vi "After Hook.vi"(8 "Error In":errorcluster, 11 "Hook VI In":path=path "") -> (0 "Error Out":errorcluster, 3 "Hook VI Out":path)   [LabVIEW 2018, in "Tests.lvlib" / "Toolkit.lvlib" / "Integration.lvlib"]
uses:
  Integration.lvlib
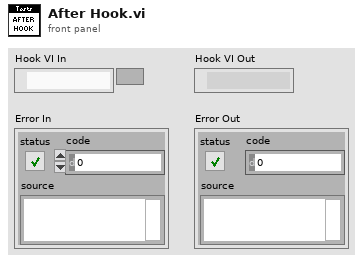
[diagram p1: front panel]
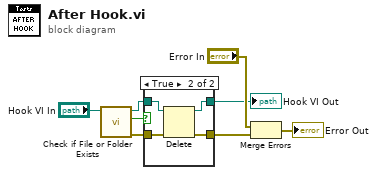
[diagram p0: block diagram]
diagram:
  n1 = call <vilib>:"Check if File or Folder Exists.vi"("path"="Hook VI In") -> ("error out"=w1:errorcluster, "file or folder exists?"=w2:bool, "dup path"=w3:path)  [unwired: 8 in]
  n2 = case shown="True" w2 {
    tunnel: [w9 w14] -> w6
    tunnel: [w10 w13] -> w5
    tunnel: w3 -> [w10 w12]
    tunnel: w1 -> [w9 w11]
    frame False {
    }
    frame True {
      n3 = Delete(path (use dialog)=w12, error in=w11) -> (deleted path=w13:path, error out=w14:errorcluster)  [unwired: 3 in, 1 out]
    }
  }
  "Hook VI Out" <- w5
  n4 = Merge Errors("Error In", w6) -> (→"Error Out":errorcluster)
